vi "Async Read Test.vi"() -> ()   [LabVIEW 2016]
panel:
  out "Data":i8[](array[numeric])
  out "Boolean":bool
  out "Sample Rate (Hz)":u32
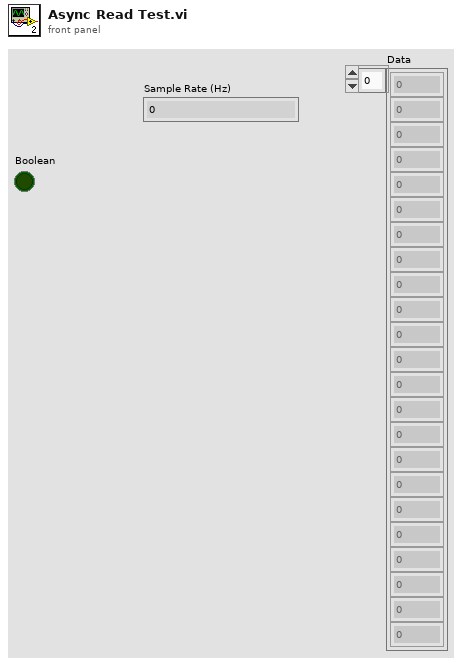
[diagram p1: front panel]
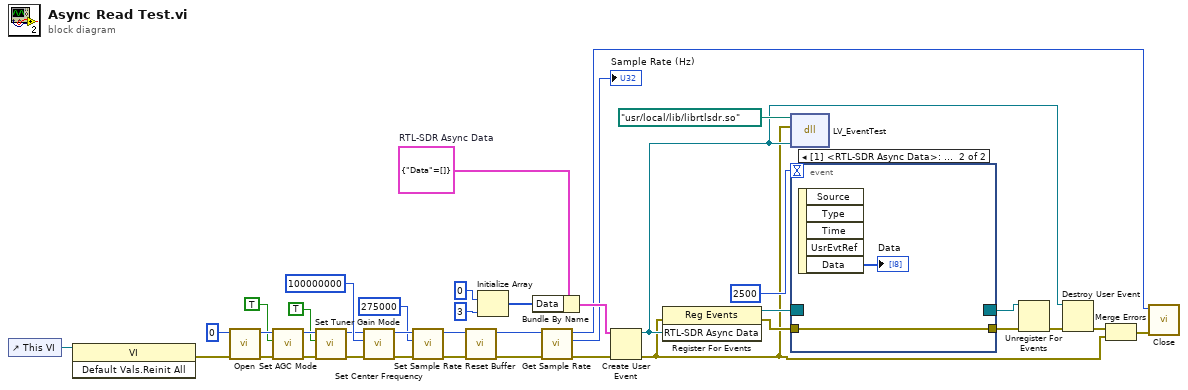
[diagram p0: block diagram]
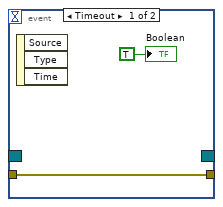
[diagram p2: hidden frame]
diagram:
  w19 = cluster{"Data":i8[]} {"Data"=[]}  # RTL-SDR Async Data
  n1 = control-ref of="This VI"() -> (w3:refnum<vi>)
  n2 = invoke class="VI" method="Default Vals.Reinit All"(reference=w3) -> (error out=w2:errorcluster)  [unwired: 2 in, 2 out]
  n3 = call "Open.vi"("error in (no error)"=w2, "Device Index"=u32 0) -> ("error out"=w25:errorcluster, "DeviceRefnum Out"=w27:u64)  [unwired: 6 in]
  n4 = call "Set AGC Mode.vi"("error in (no error)"=w25, "AGC Enable"=TRUE, "DeviceRefnum"=w27) -> ("error out"=w24:errorcluster, "DeviceRefnum Out"=w26:u64)  [unwired: 6 in, 1 out]
  n5 = call "Set Tuner Gain Mode.vi"("error in (no error)"=w24, "AutoGain"=TRUE, "DeviceRefnum"=w26) -> ("error out"=w22:errorcluster, "DeviceRefnum Out"=w23:u64)  [unwired: 6 in, 1 out]
  n6 = call "Set Center Frequency.vi"("error in (no error)"=w22, "Center Frequency"=u32 100000000, "DeviceRefnum"=w23) -> ("error out"=w31:errorcluster, "DeviceRefnum Out"=w32:u64)  [unwired: 6 in, 1 out]
  n7 = call "Set Sample Rate.vi"("error in (no error)"=w31, "Sample Rate"=u32 275000, "DeviceRefnum"=w32) -> ("error out"=w29:errorcluster, "DeviceRefnum Out"=w30:u64)  [unwired: 6 in, 1 out]
  n8 = call "Reset Buffer.vi"("error in (no error)"=w29, "DeviceRefnum"=w30) -> ("error out"=w13:errorcluster, "DeviceRefnum Out"=w11:u64)  [unwired: 7 in, 1 out]
  n9 = Initialize Array(i8 0, 3 ("dimension size")) -> (w4:i8[])
  n10 = Bundle By Name(cluster=w19, "Data"=w4) -> (w18:cluster{"Data":i8[]})
  n11 = call "Get Sample Rate.vi"("error in (no error)"=w13, "DeviceRefnum"=w11) -> ("error out"=w12:errorcluster, "Sample Rate (Hz)"=→"Sample Rate (Hz)":u32, "DeviceRefnum Out"=w10:u64)  [unwired: 7 in]
  n12 = Create User Event(user event datatype=w18, error in=w12) -> (user event=w7:refnum<user-event>, error out=w1:errorcluster)
  n13 = register-events(error in=w1, w7) -> (reference out=w16:refnum<event-registration>, error out=w14:errorcluster)  [unwired: 1 in]
  n14 = dll-call lib="usr/local/lib/librtlsdr.so" fn="LV_EventTest"(path in=path "/usr/local/lib/librtlsdr.so", error in=w1, "msg"=w7) -> ()  [unwired: 3 in, 2 out]
  n15 = event shown="[1] <RTL-SDR Async Data>: User Event" {
    selector: w16 -> [_ _]
    dyn-events: [_ _] -> w15
    timeout: 2500 -> [_ _]
    tunnel: [w39 w42] -> w17
    tunnel: w14 -> [w39 w42]
    event Timeout {
      n16 = event-data() -> ()  [unwired: 1 in, 3 out]
      "Boolean" <- TRUE ("Boolean")
    }
    event User Event {
      n17 = event-data() -> ("Data"=→"Data":i8[])  [unwired: 1 in, 4 out]
    }
  }
  n18 = Unregister For Events(event registration refnum=w15, error in=w17) -> (error out=w35:errorcluster)
  n19 = Destroy User Event(user event=w7, error in=w35) -> (error out=w34:errorcluster)
  n20 = Merge Errors(w34, w1) -> (w33:errorcluster)
  n21 = call "Close.vi"("error in (no error)"=w33, "DeviceRefnum"=w10) -> ()  [unwired: 8 in, 2 out]
